vi "hw3p8_hickey.vi"() -> ()   [LabVIEW 2014]
uses:
  <vilib>/Analysis/baseanly.llb/Mean (DBL).vi
  <vilib>/Analysis/NI_AALBase.lvlib
panel:
  out "Average":dbl
  out "Array":i32[](array[numeric])
  in  "N":i32
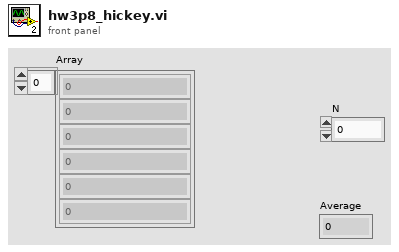
[diagram p1: front panel]
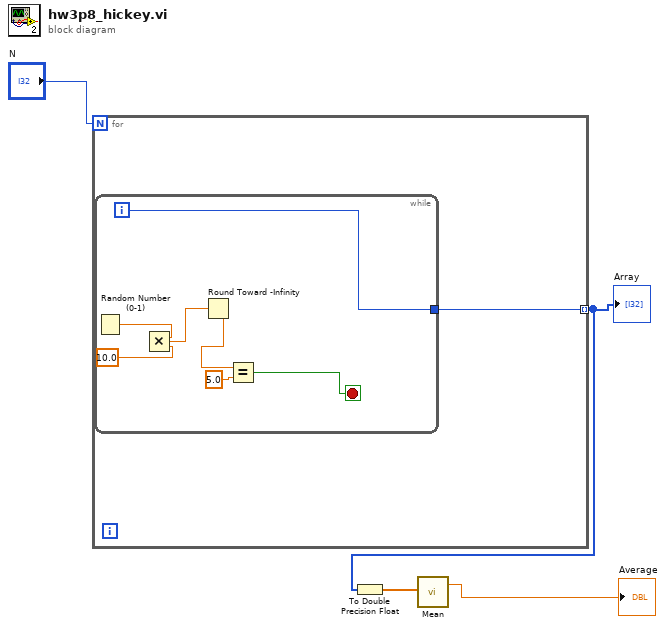
[diagram p0: block diagram]
diagram:
  n1 = for {
    N: "N" -> [_]
    tunnel: [w5] -> w2 mode=indexing
    n2 = while {
      tunnel: [w6] -> w5
      i -> [w6]
      stop <- w9 stop-if-true
      n3 = Random Number (0-1)() -> (number: 0 to 1=w12:dbl)
      n4 = Multiply(x=w12, y=10.0) -> (x*y=w8:dbl)
      n5 = Round Toward -Infinity(1:w8) -> (0:w7:dbl)
      n6 = Equal?(x=w7, y=5.0) -> (x = y?=w9:bool)
    }
  }
  "Array" <- w2
  n7 = To Double Precision Float(number=w2) -> (double precision float=w1:dbl[])
  n8 = call-poly <vilib>:"Mean.vi"("X"=w1) -> ("mean"=→"Average":dbl)  [unwired: 1 out]
